vi "PopulateRings.vi"(8 "error in (no error)":errorcluster, 11 "MAUI in":refnum<class "SMO.UI.MAUI.lvclass">) -> (0 "error out":errorcluster, 3 "MAUI out":refnum<class "SMO.UI.MAUI.lvclass">)   [LabVIEW 2020, in "SMO.UI.MAUI.lvclass"]
uses:
  SMO.UI.MAUI.lvclass
  SMO.UI.MAUI.lvclass/SMO.UI.MAUI.ctl
  <vilib>/Levylab/SMO.UI.Embedded/SMO.UI.Embedded.lvclass
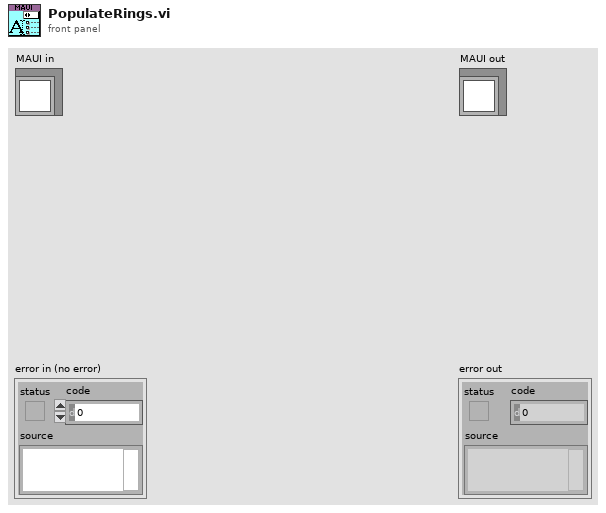
[diagram p1: front panel]
types:
  T1 = typedef "SMO.UI.MAUI.lvclass/PanelData.ctl" = cluster{"SubPanel":refnum<vi>, "Ring":refnum<vi>, "Active":i32}
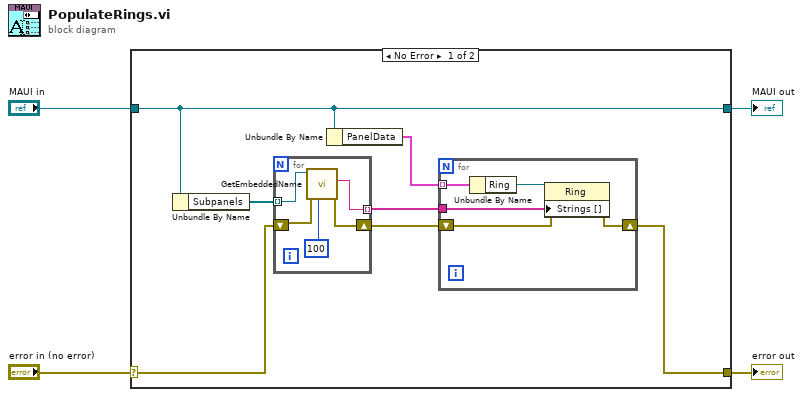
[diagram p0: block diagram]
diagram:
  n1 = case shown="No Error" "error in (no error)" {
    selector: "error in (no error)" -> [w9 w23]
    tunnel: [w5 w23] -> w3
    tunnel: [w11 w22] -> w1
    tunnel: "MAUI in" -> [w11 w22]
    frame No Error {
      n2 = Unbundle By Name(w11) -> ("Subpanels"=w10:refnum<class "SMO.UI.Embedded.lvclass">[])
      n3 = for {
        tunnel: w10 -> [w21] mode=indexing
        tunnel: [w20] -> w7 mode=indexing
        shift-right: [w19] -> w6
        shift-left: w9 -> [w18]
        n4 = call <vilib>:"GetEmbeddedName.vi"("timeout in ms (-1)"=100, "error in (no error)"=w18, "EmbeddedSMO in"=w21) -> ("error out"=w19:errorcluster, "Name"=w20:string)  [unwired: 6 in, 1 out]
      }
      n5 = Unbundle By Name(w11) -> ("PanelData"=w8:T1[])
      n6 = for {
        tunnel: w8 -> [w16] mode=indexing
        tunnel: w7 -> [w14]
        shift-right: [w12] -> w5
        shift-left: w6 -> [w13]
        n7 = Unbundle By Name(w16) -> ("Ring"=w15:refnum<vi>)
        n8 = property class="Ring"(reference=w15, error in=w13, "Strings []"=w14) -> (error out=w12:errorcluster)  [unwired: 1 out]
      }
    }
    frame Error {
    }
  }
  "error out" <- w3
  "MAUI out" <- w1
